vi "iWorx - Pulse.vi"() -> ()   [LabVIEW 2012]
uses:
  <vilib>/DAQmx/read.llb/DAQmx Read (Analog 1D Wfm NChan NSamp).vi
  <vilib>/DAQmx/create/channels.llb/DAQmx Create Channel (AI-Voltage-Basic).vi
  <vilib>/DAQmx/configure/timing.llb/DAQmx Timing (Sample Clock).vi
  <vilib>/measure/macond.llb/IIR Filter for 1 Chan.vi
  <vilib>/DAQmx/miscellaneous.llb/DAQmx Fill In Error Info.vi
  <vilib>/measure/NI_MAPro.lvlib
panel:
  out "Heart Signal":waveform(dbl)(graph)
  out "Avg Pulse":dbl format="%5.1f BPM"
  out "Inst Pulse":dbl format="%5.1f BPM"
  in  "Threshold":dbl=0.0005 step=0.0001 format="%_3p"
  in  "Calibrate":bool
  out "error out":errorcluster
  in  "Set Up":bool
  in  "Channel":u16(ring) items=["Channel 1", "Channel 2"]
  in  "Pause Button":bool
  in  "Snapshot":bool
  in  "stop":bool
  in  "Clear Chart":bool
  in  "Open Log":bool
  in  "Autoscale Y":bool
  out "Raw Signal":dbl(knob) scale=-1.0..1.0
  # "iWorx - Pulse - Data Logger"
  # "Sensor Input"
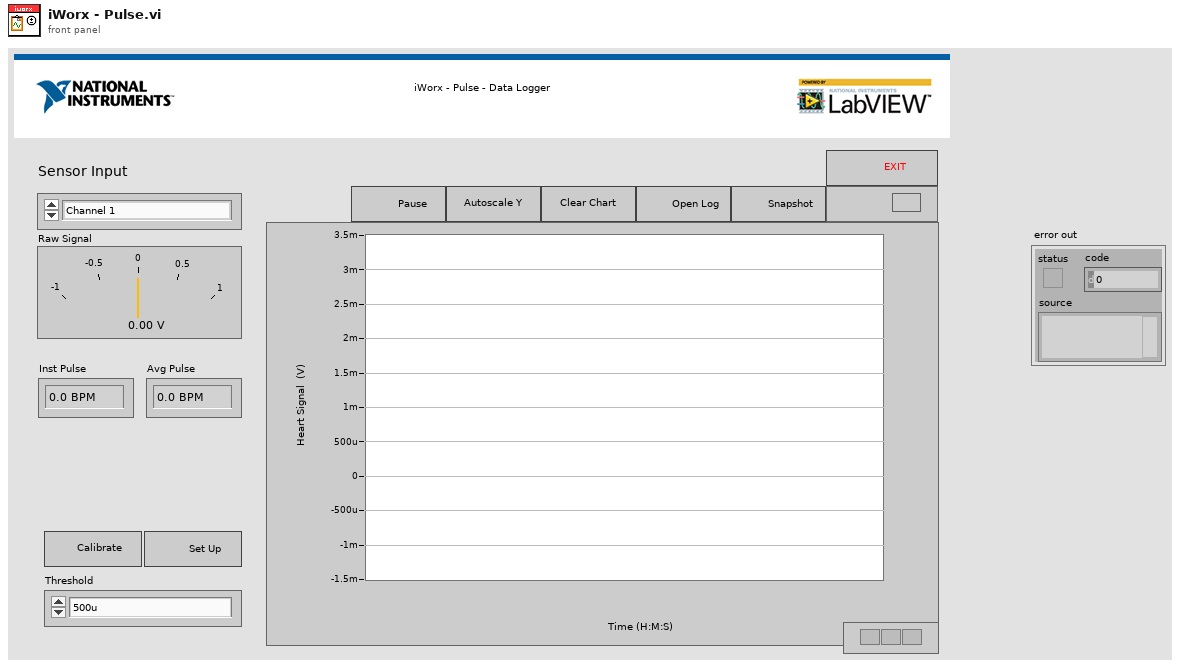
[diagram p1: front panel]
types:
  T1 = cluster{"Topology":enum16{"Off", "Butterworth", "Chebyshev", "Inverse Chebyshev", "Elliptic", "Bessel"}, "Type":enum16{"Lowpass", "Highpass", "Bandpass", "Bandstop"}, "Order":i32, "Lower Fc":dbl, "Upper Fc":dbl, "PB Ripple":dbl, "SB Attenuation":dbl}
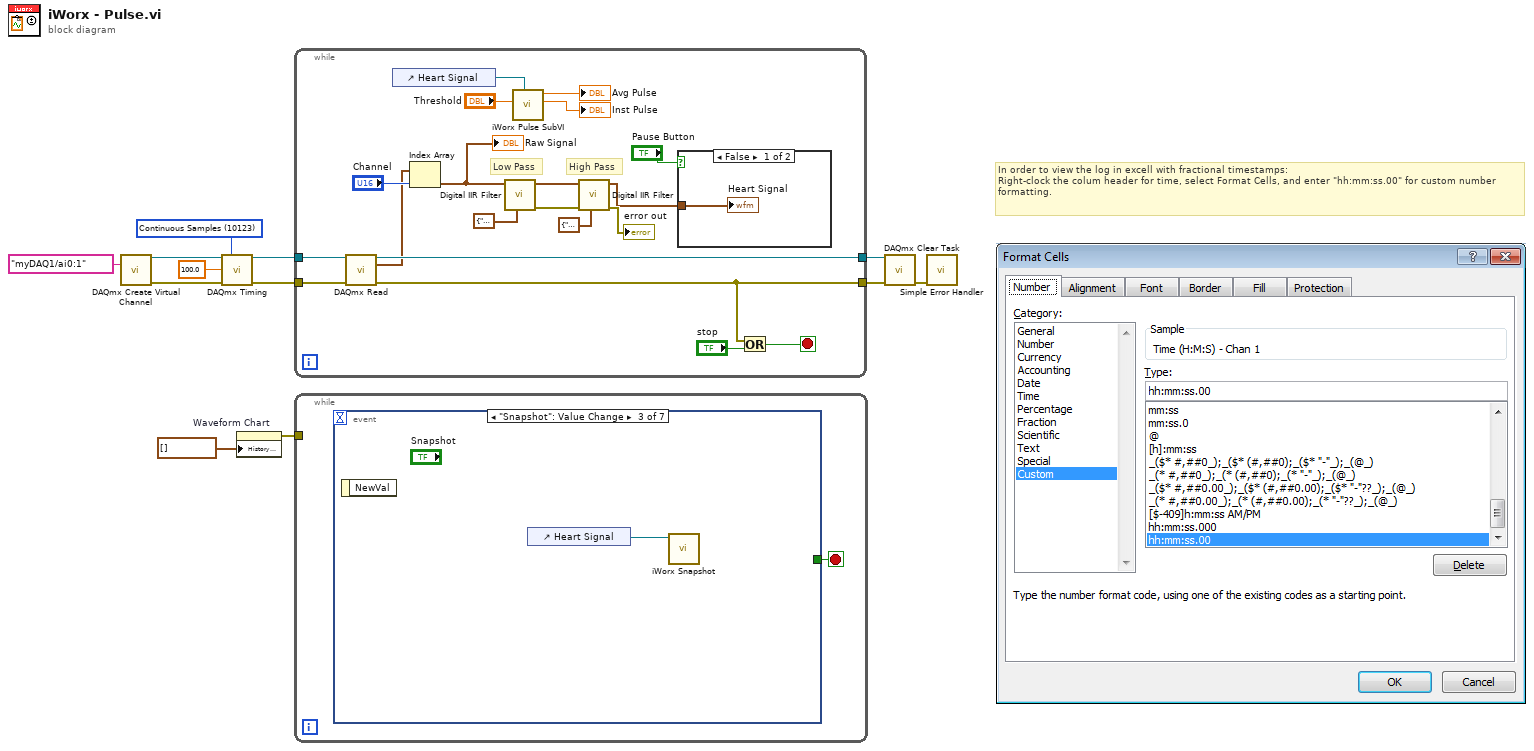
[diagram p0: block diagram]
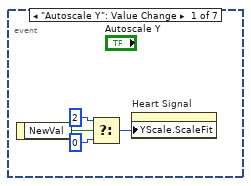
[diagram p2: hidden frame]
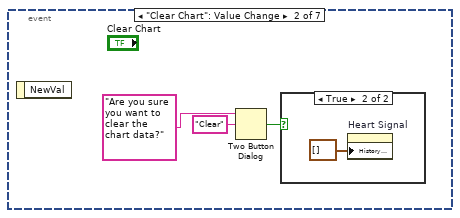
[diagram p3: hidden frame]
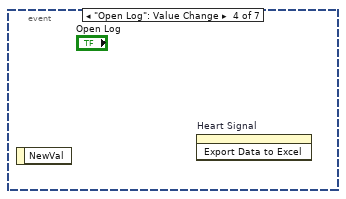
[diagram p5: hidden frame]
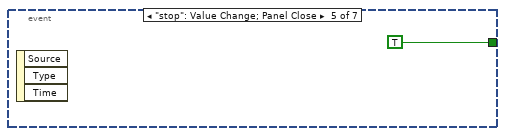
[diagram p6: hidden frame]
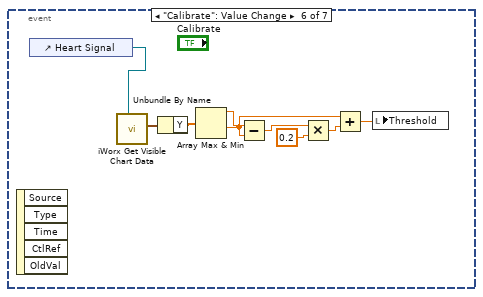
[diagram p7: hidden frame]
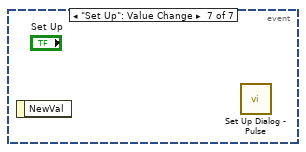
[diagram p8: hidden frame]
diagram:
  w2 = 10123 items=["Finite Samples"=10178, "Continuous Samples"=10123, "Hardware Timed Single Point"=12522] ("sample mode")
  # "In order to view the log in excell with fractional timestamps: \nRight-clock the colum header for time, select Format Cells, and enter \"hh:mm:ss.00\" for custom number formatting."
  n1 = call-poly <vilib>:"DAQmx Create Virtual Channel.vi"("physical channels"=tag "myDAQ1/ai0:1") -> ("task out"=w6:refnum<k21>, "error out"=w5:errorcluster)  [unwired: 13 in]
  n2 = call-poly <vilib>:"DAQmx Timing.vi"("task/channels in"=w6, "sample mode"=w2, "rate"=100.0, "error in"=w5) -> ("task out"=w3:refnum<k21>, "error out"=w4:errorcluster)  [unwired: 10 in]
  n3 = property on="Waveform Chart" class="WFChart (strict)"("History Data"=waveform(dbl)[] []) -> (error out=w7:errorcluster)  [unwired: 2 in, 1 out]
  n4 = while {
    tunnel: w3 -> [w31]
    tunnel: [w30] -> w12
    tunnel: w4 -> [w29]
    tunnel: [w27] -> w11
    stop <- w28 stop-if-true
    # "High Pass"
    # "Low Pass"
    n5 = call-poly <vilib>:"DAQmx Read.vi"("task/channels in"=w31, "error in"=w29) -> ("task out"=w30:refnum<k21>, "data"=w24:waveform(dbl)[], "error out"=w27:errorcluster)  [unwired: 11 in]
    n6 = control-ref of="Heart Signal"() -> (w17:refnum<vi>)
    n7 = Index Array(array=w24, index="Channel") -> (element=w15:waveform(dbl))
    "Raw Signal" <- w15
    n8 = call-poly <vilib>:"Digital IIR Filter.vi"("IIR filter specifications"=T1 {"Topology"=enum."Butterworth", "Type"=enum."Lowpass", "Order"=1, "Lower Fc"=0.001, "Upper Fc"=200.0, "PB Ripple"=1.0, "SB Attenuation"=60.0}, "signal in"=w15) -> ("error out"=w21:errorcluster, "signal out"=w18:waveform(dbl))  [unwired: 7 in, 1 out]
    n9 = call "iWorx Pulse SubVI.vi"("Pulse Chart"=w17, "Threshold (.5mV)"="Threshold") -> ("Inst Pulse Rate (BPM)"=→"Inst Pulse":dbl, "Average Pulse Rate (BPM)"=→"Avg Pulse":dbl)  [unwired: 7 in, 1 out]
    n10 = call-poly <vilib>:"Digital IIR Filter.vi"("IIR filter specifications"=T1 {"Topology"=enum."Butterworth", "Type"=enum."Highpass", "Order"=1, "Lower Fc"=1.0, "Upper Fc"=10.0, "PB Ripple"=1.0, "SB Attenuation"=60.0} ("IIR filter specifications 2"), "error in (no error)"=w21, "signal in"=w18) -> ("error out"=→"error out":errorcluster, "signal out"=w20:waveform(dbl))  [unwired: 6 in, 1 out]
    n11 = case shown="False" "Pause Button" {
      tunnel: w20 -> [w33 _]
      frame False {
        "Heart Signal" <- w33
      }
      frame True {
      }
    }
    n12 = Or(x=w27, y="stop") -> (x .or. y?=w28:bool)
  }
  n13 = while {
    tunnel: w7 -> [_]
    stop <- w34 stop-if-true
    n14 = event shown="[2] \"Snapshot\": Value Change" {
      selector: _ -> [_ _ _ _ _ _ _]
      dyn-events: _ -> [_ _ _ _ _ _ _]
      timeout: _ -> [_ _ _ _ _ _ _]
      tunnel: [_ _ _ _ TRUE _ _] -> w34
      event "Autoscale Y": Value Change {
        n15 = event-data() -> ("NewVal"=w36:bool)  [unwired: 1 in]
        n16 = Select(t=u8 2 ("Y Scale.Scale Fit"), s=w36, f=u8 0 ("Y Scale.Scale Fit")) -> (s? t:f=w35:u8)
        n17 = property on="Heart Signal" class="WFChart (strict)"("YScale.ScaleFit"=w35) -> ()  [unwired: 2 in, 2 out]
      }
      event "Clear Chart": Value Change {
        n18 = event-data() -> ()  [unwired: 1 in, 1 out]
        n19 = Two Button Dialog(message="Are you sure you want to clear the chart data?", 2:"Clear" ("T button name (\"OK\")")) -> (T button?=w40:bool)  [unwired: 1 in]
        n20 = case shown="True" w40 {
          frame False {
          }
          frame True {
            n21 = property on="Heart Signal" class="WFChart (strict)"("History Data"=waveform(dbl)[] []) -> ()  [unwired: 2 in, 2 out]
          }
        }
      }
      event "Snapshot": Value Change {
        n22 = event-data() -> ()  [unwired: 1 in, 1 out]
        n23 = control-ref of="Heart Signal"() -> (w43:refnum<vi>)
        n24 = call "iWorx Snapshot.vi"("WaveformChart in"=w43) -> ()  [unwired: 10 in, 1 out]
      }
      event "Open Log": Value Change {
        n25 = event-data() -> ()  [unwired: 1 in, 1 out]
        n26 = invoke on="Heart Signal" class="WFChart (strict)" method="Export Data to Excel"() -> ()  [unwired: 3 in, 3 out]
      }
      event "stop": Value Change; Panel Close {
        n27 = event-data() -> ()  [unwired: 1 in, 3 out]
      }
      event "Calibrate": Value Change {
        n28 = event-data() -> ()  [unwired: 1 in, 5 out]
        n29 = control-ref of="Heart Signal"() -> (w52:refnum<vi>)
        n30 = call "iWorx Get Visible Chart Data.vi"("Selection Chart"=w52) -> ("waveform out"=w53:waveform(dbl))  [unwired: 8 in, 2 out]
        n31 = Unbundle By Name(w53) -> ("Y"=w46:dbl[])
        n32 = Array Max & Min(array=w46) -> (max value=w47:dbl, min value=w51:dbl)  [unwired: 2 out]
        n33 = Subtract(x=w47, y=w51) -> (x-y=w48:dbl)
        n34 = Multiply(x=w48, y=0.2) -> (x*y=w50:dbl)
        n35 = Add(x=w51, y=w50) -> (x+y=w45:dbl)
        n36 = local write "Threshold"(w45) -> ()
      }
      event "Set Up": Value Change {
        n37 = event-data() -> ()  [unwired: 1 in, 1 out]
        n38 = call "Set Up Dialog - Pulse.vi"() -> ()  [unwired: 12 in]
      }
    }
  }
  n39 = call <vilib>:"DAQmx Clear Task.vi"("task in"=w12, "error in"=w11) -> ("error out"=w9:errorcluster)  [unwired: 13 in]
  n40 = call <vilib>:"Simple Error Handler.vi"("error in (no error)"=w9) -> ()  [unwired: 4 in, 5 out]
